vi "Smista AO.vi"(0 "AO scalati IN":T3, 9 "Forza AO plc_3":T1, 12 "Forza AO cdaq":T2) -> (4 "statoAO_Cdaq out":T2, 15 "statoAO_PLC 3 out":T1)   [LabVIEW 2019]
uses:
  cDAQ_PLC Folder/controls/StatoAO_cdaq.ctl
  TypeDef/Lista AO sistema.ctl
  cDAQ_PLC Folder/controls/statoAO_plc_3.ctl
  GlobalForzaUscite.vi
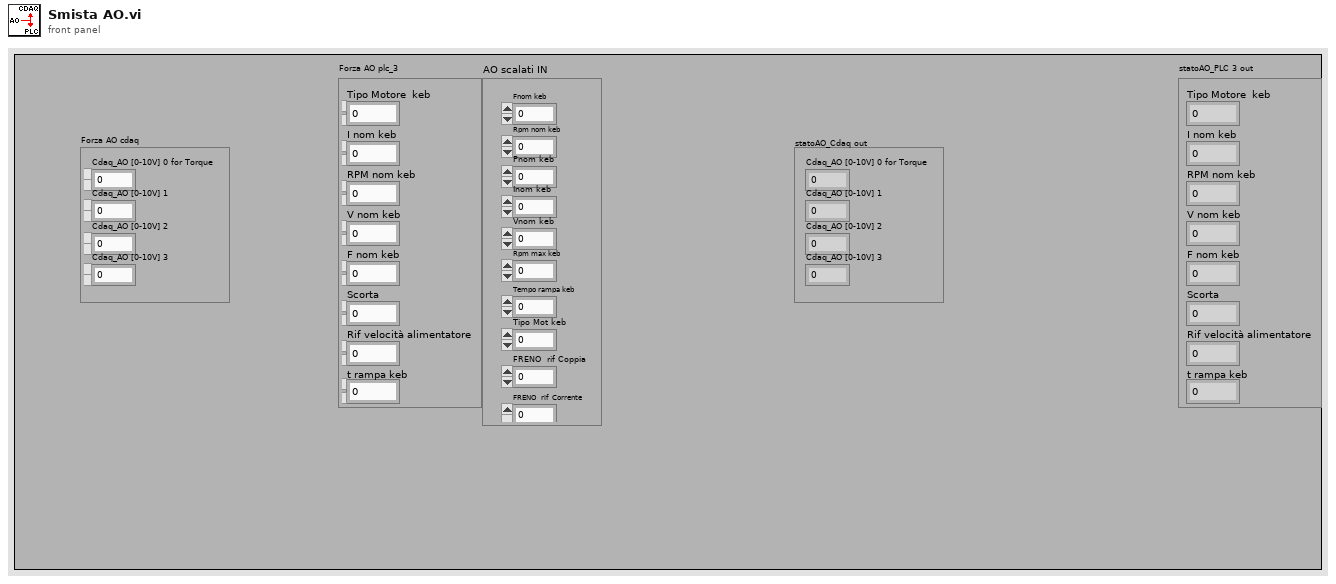
[diagram p1: front panel]
types:
  T1 = typedef "statoAO_plc_3.ctl" = cluster{"Rif velocità alimentatore":dbl, "Scorta":dbl, "Tipo Motore  keb":dbl, "I nom keb":dbl, "RPM nom keb":dbl, "V nom keb":dbl, "F nom keb":dbl, "t rampa keb":dbl}
  T2 = typedef "StatoAO_cdaq.ctl" = cluster{"Cdaq_AO [0-10V] 0 for Torque":dbl, "Cdaq_AO [0-10V] 1":dbl, "Cdaq_AO [0-10V] 2":dbl, "Cdaq_AO [0-10V] 3":dbl}
  T3 = typedef "Lista AO sistema.ctl" = cluster{"FRENO1 rif vel":dbl, "FRENO1 rif Coppia":dbl, "FRENO2 rif vel":dbl, "FRENO2 rif Coppia":dbl, "ALIM1 rif V":dbl, "ALIM1 rif F":dbl, "ALIM2 rif V":dbl, "ALIM2 rif F":dbl, "ALIM3 rif V":dbl, "ALIM3 rif F":dbl, "Fnom keb":dbl, "Rpm nom keb":dbl, "Pnom keb":dbl, "Inom keb":dbl, "Vnom keb":dbl, "Rpm max keb":dbl, "Tempo rampa keb":dbl, "Tipo Mot keb":dbl, "FRENO  rif Coppia ":dbl, "FRENO  rif  Corrente":dbl}
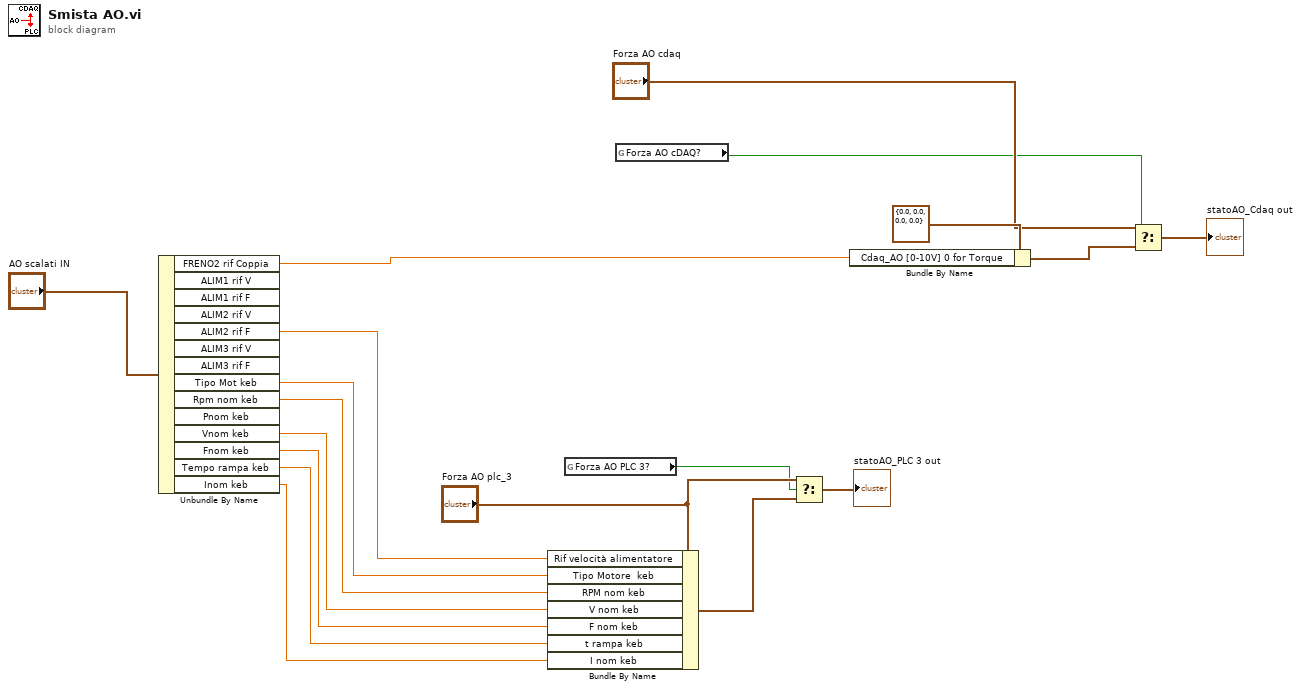
[diagram p0: block diagram]
diagram:
  n1 = Unbundle By Name("AO scalati IN") -> ("FRENO2 rif Coppia"=w1:dbl, "ALIM2 rif F"=w2:dbl, "Tipo Mot keb"=w8:dbl, "Rpm nom keb"=w7:dbl, "Vnom keb"=w6:dbl, "Fnom keb"=w5:dbl, "Tempo rampa keb"=w4:dbl, "Inom keb"=w3:dbl)  [unwired: 6 out]
  n2 = Bundle By Name(cluster="Forza AO plc_3", "Rif velocità alimentatore"=w2, "Tipo Motore  keb"=w8, "RPM nom keb"=w7, "V nom keb"=w6, "F nom keb"=w5, "t rampa keb"=w4, "I nom keb"=w3) -> (w13:T1)
  n3 = global read "GlobalForzaUscite.vi" "Forza AO PLC 3?"() -> (w9:bool)
  n4 = global read "GlobalForzaUscite.vi" "Forza AO cDAQ?"() -> (w10:bool)
  n5 = Select(t="Forza AO plc_3", s=w9, f=w13) -> (s? t:f=→"statoAO_PLC 3 out":T1)
  n6 = Bundle By Name(cluster=T2 {"Cdaq_AO [0-10V] 0 for Torque"=0.0, "Cdaq_AO [0-10V] 1"=0.0, "Cdaq_AO [0-10V] 2"=0.0, "Cdaq_AO [0-10V] 3"=0.0} ("statoAO_Cdaq out"), "Cdaq_AO [0-10V] 0 for Torque"=w1) -> (w16:T2)
  n7 = Select(t="Forza AO cdaq", s=w10, f=w16) -> (s? t:f=→"statoAO_Cdaq out":T2)
